vi "start waveform.vi"(4 "length":u16, 5 "time":dbl, 6 "trig_level":u32, 7 "trig_mask":u32, 8 "error in (no error)":errorcluster, 9 "dec_ratio":u16, 10 "mode":u16, 11 "identifier":string) -> (0 "error out":errorcluster, 3 "function return":u32)   [LabVIEW 2015, in "XGL_DPP.lvlib"]
doc: "EXTERN DECLSPEC unsigned int CALL_CONV start_waveform(const char* identifier,\n unsigned short int mode,\n unsigned short int dec_ratio,\n unsigned int trig_mask,\n unsigned int trig_level,\n const double time,\n unsigned short int length);"
uses:
  XGL_DPP.lvlib
  D:/Scanning Software_Demokritos_2015_v6/libs/XGL_DPP.dll
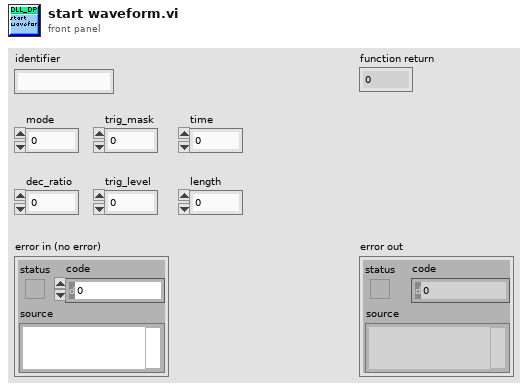
[diagram p1: front panel]
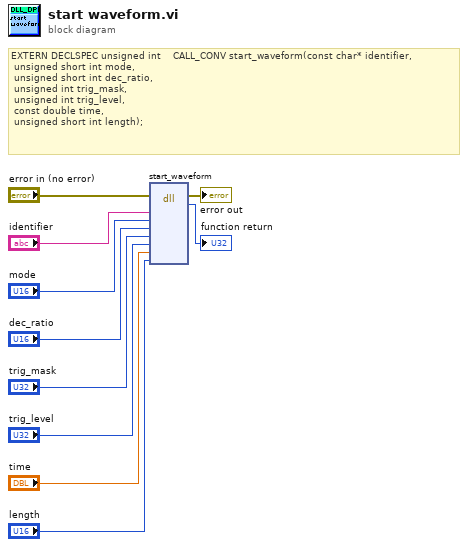
[diagram p0: block diagram]
diagram:
  # "EXTERN DECLSPEC unsigned int    CALL_CONV start_waveform(const char* identifier,\n unsigned short int mode,\n unsigned short int dec_ratio,\n unsigned int trig_mask,\n unsigned int trig_level,\n const double time,\n unsigned short int length);"
  n1 = dll-call lib="D:/Scanning Software_Demokritos_2015_v6/libs/XGL_DPP.*" fn="start_waveform"(error in="error in (no error)", "identifier"="identifier", "mode"="mode", "dec_ratio"="dec_ratio", "trig_mask"="trig_mask", "trig_level"="trig_level", "time"="time", "length"="length") -> (error out=→"error out":errorcluster, "return type"=→"function return":u32)  [unwired: 9 in, 1 out]
